vi "9_Compensate_Input_Delays_setInputDelay.vi"(8 "error in (no error)":errorcluster) -> (0 "error out":errorcluster)   [LabVIEW 2014]
uses:
  SwabianInstruments.TimeTagger
panel:
  in  "Clear Data":bool
  out "Counts per second":dbl[](array[numeric])
  in  "End Measurement":bool
  out "Rate":dbl[](array[numeric]) caption="Counts/s with delay adjustment"
  out "extracted delay [ps]\n (peak maximum)":i64
  out "Cross correlation":cluster{"getIndex":i64[], "getData":i32[]}(graph) caption="Cross correlation with compensated delay"
  out "Cross correlation without inputDelay adjustment":cluster{"getIndex":i64[], "getData":i32[]}(graph)
  # "STAGE 1\nThe internal test signal has a propagation delay between the \ndifferent input channels.\nThis example shows how to use setInputDelay to compensate the offset."
  # "STAGE 2\nThe internal test signal of channel 1 is now shifted from the measurement\nof STAGE 1 so that clicks of both channels arrive at the very same time."
  # "channel 1"
  # "channel 1"
  # "channel 2"
  # "channel 2"
  # "coincidences"
  # "coincidences"
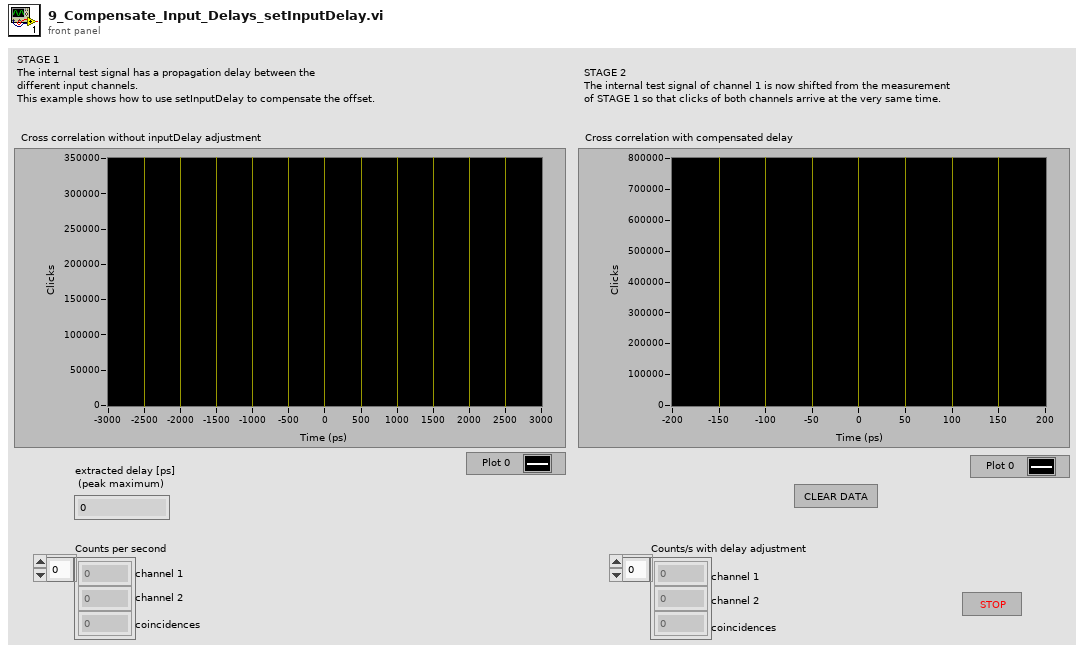
[diagram p1: front panel]
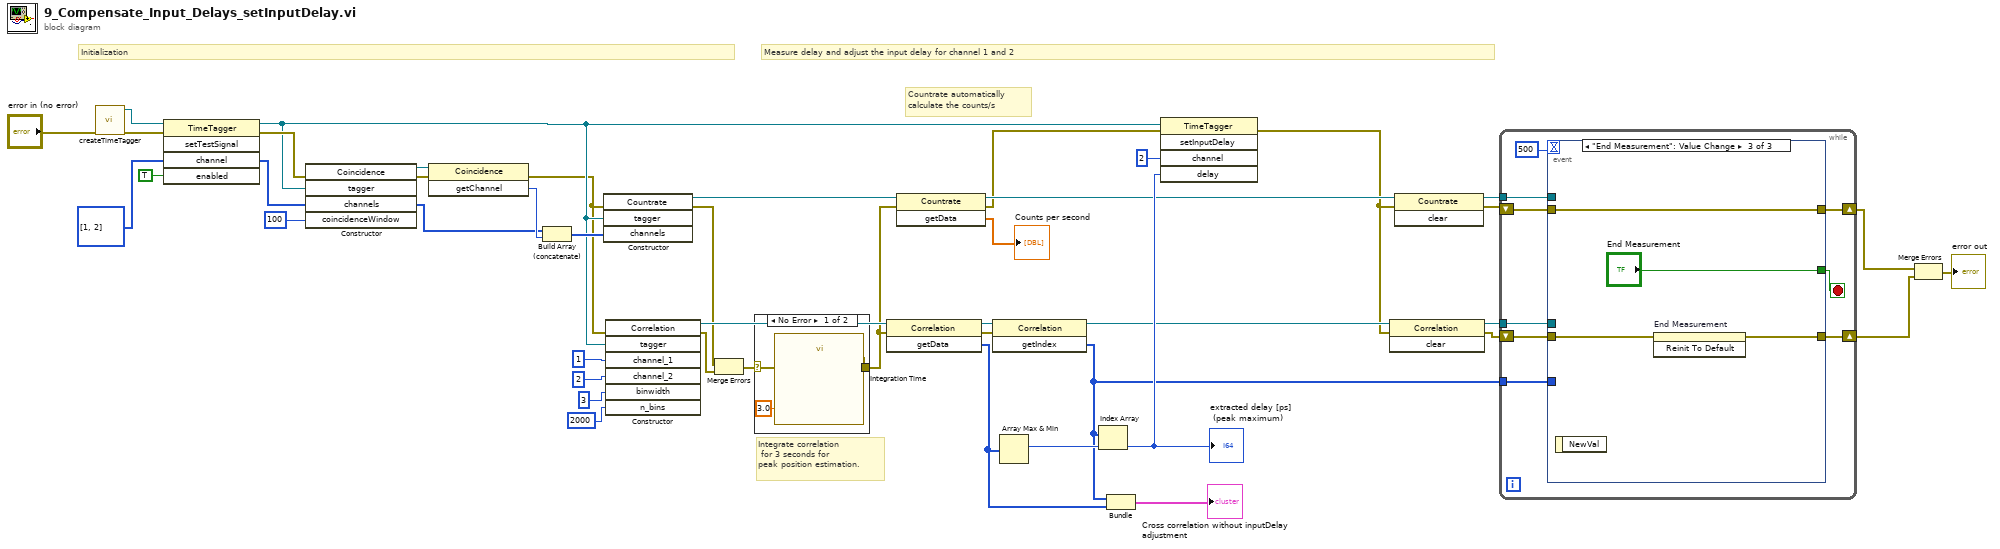
[diagram p0: block diagram]
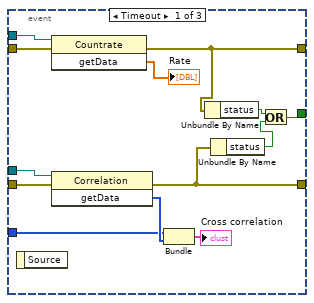
[diagram p3: hidden frame]
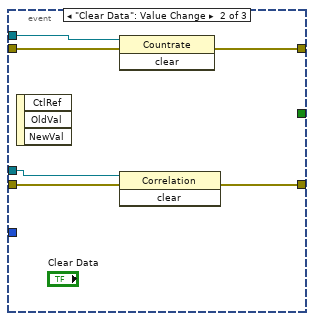
[diagram p4: hidden frame]
diagram:
  # "Integrate correlation\n for 3 seconds for\npeak position estimation."
  # "Countrate automatically \ncalculate the counts/s"
  # "Measure delay and adjust the input delay for channel 1 and 2"
  # "Initialization"
  n1 = call "createTimeTagger.vi"("error in (no error)"="error in (no error)") -> ("error out"=w19:errorcluster, "TimeTagger ref out"=w18:refnum<k24>)  [unwired: 9 in]
  n2 = invoke class="TimeTagger" method="setTestSignal"(reference=w18, error in=w19, "channel"=i32[] [1, 2], "enabled"=TRUE) -> (reference out=w7:refnum<k24>, error out=w16:errorcluster, "channel"=w13:i32[])  [unwired: 1 in, 2 out]
  n3 = constructor class="Coincidence"(error in=w16, "tagger"=w7, "channels"=w13, "coincidenceWindow"=i64 100 ("window")) -> (reference out=w22:refnum<k24>, error out=w20:errorcluster, "channels"=w14:i32[])  [unwired: 2 in, 3 out]
  n4 = invoke class="Coincidence" method="getChannel"(reference=w22, error in=w20) -> (error out=w6:errorcluster, "getChannel"=w21:i32)  [unwired: 1 in, 1 out]
  n5 = Build Array (concatenate)(w14, w21) -> (w33:i32[])
  n6 = constructor class="Countrate"(error in=w6, "tagger"=w7, "channels"=w33) -> (reference out=w26:refnum<k24>, error out=w10:errorcluster)  [unwired: 2 in, 3 out]
  n7 = constructor class="Correlation"(error in=w6, "tagger"=w7, "channel_1"=1, "channel_2"=2, "binwidth"=i64 3, "n_bins"=2000) -> (reference out=w30:refnum<k24>, error out=w9:errorcluster)  [unwired: 2 in, 6 out]
  n8 = Merge Errors(w10, w9) -> (w8:errorcluster)
  n9 = case shown="No Error" w8 {
    selector: w8 -> [w46 w49]
    tunnel: [w47 w49] -> w15
    frame No Error {
      n10 = call "Integration Time"("error in (no error)"=w46, "Delay Time (s)"=3.0) -> ("error out"=w47:errorcluster)  [unwired: 9 in]
    }
    frame Error {
    }
  }
  n11 = invoke class="Correlation" method="getData"(reference=w30, error in=w15) -> (reference out=w44:refnum<k24>, error out=w27:errorcluster, "getData"=w38:i32[])  [unwired: 1 in]
  n12 = invoke class="Countrate" method="getData"(reference=w26, error in=w15) -> (reference out=w25:refnum<k24>, error out=w23:errorcluster, "getData"=→"Counts per second":dbl[])  [unwired: 1 in]
  n13 = invoke class="Correlation" method="getIndex"(reference=w44, error in=w27) -> (reference out=w31:refnum<k24>, "getIndex"=w32:i64[])  [unwired: 1 in, 1 out]
  n14 = Array Max & Min(array=w38) -> (max index (indices)=w36:i32)  [unwired: 3 out]
  n15 = Index Array(array=w32, index=w36) -> (element=w35:i64)
  "extracted delay [ps]\n (peak maximum)" <- w35
  n16 = Bundle("getIndex"=w32, "getData"=w38) -> (→"Cross correlation without inputDelay adjustment":cluster{"getIndex":i64[], "getData":i32[]})  [unwired: 1 in]
  n17 = invoke class="TimeTagger" method="setInputDelay"(reference=w7, error in=w23, "channel"=2, "delay"=w35) -> (error out=w5:errorcluster)  [unwired: 1 in, 4 out]
  n18 = invoke class="Correlation" method="clear"(reference=w31, error in=w5) -> (reference out=w29:refnum<k24>, error out=w11:errorcluster)  [unwired: 1 in, 1 out]
  n19 = invoke class="Countrate" method="clear"(reference=w25, error in=w5) -> (reference out=w28:refnum<k24>, error out=w12:errorcluster)  [unwired: 1 in, 1 out]
  n20 = while {
    tunnel: w32 -> [w58]
    tunnel: w29 -> [w57]
    tunnel: w28 -> [w56]
    shift-right: [w53] -> w3
    shift-left: w11 -> [w55]
    shift-right: [w52] -> w4
    shift-left: w12 -> [w54]
    stop <- w51 stop-if-true
    n21 = event shown="[2] \"End Measurement\": Value Change" {
      selector: _ -> [_ _ _]
      dyn-events: _ -> [_ _ _]
      timeout: u32 500 ("milliseconds to wait") -> [_ _ _]
      tunnel: w58 -> [w70 _ _]
      tunnel: w57 -> [w68 w75 _]
      tunnel: w56 -> [w67 w77 _]
      tunnel: w55 -> [w65 w74 w79]
      tunnel: w54 -> [w64 w76 w80]
      tunnel: [w63 w73 w78] -> w53
      tunnel: [w62 w72 w80] -> w52
      tunnel: [w59 _ "End Measurement"] -> w51
      event Timeout {
        n22 = event-data() -> ()  [unwired: 1 in, 1 out]
        n23 = invoke class="Countrate" method="getData"(reference=w67, error in=w64) -> (error out=w62:errorcluster, "getData"=→"Rate":dbl[])  [unwired: 1 in, 1 out]
        n24 = invoke class="Correlation" method="getData"(reference=w68, error in=w65) -> (error out=w63:errorcluster, "getData"=w71:i32[])  [unwired: 1 in, 1 out]
        n25 = Bundle("getIndex"=w70, "getData"=w71) -> (→"Cross correlation":cluster{"getIndex":i64[], "getData":i32[]})  [unwired: 1 in]
        n26 = Unbundle By Name(w62) -> ("status"=w61:bool)
        n27 = Unbundle By Name(w63) -> ("status"=w60:bool)
        n28 = Or(x=w61, y=w60) -> (x .or. y?=w59:bool)
      }
      event "Clear Data": Value Change {
        n29 = event-data() -> ()  [unwired: 1 in, 3 out]
        n30 = invoke class="Countrate" method="clear"(reference=w77, error in=w76) -> (error out=w72:errorcluster)  [unwired: 1 in, 2 out]
        n31 = invoke class="Correlation" method="clear"(reference=w75, error in=w74) -> (error out=w73:errorcluster)  [unwired: 1 in, 2 out]
      }
      event "End Measurement": Value Change {
        n32 = event-data() -> ()  [unwired: 1 in, 1 out]
        n33 = invoke on="End Measurement" class="Bool (strict)" method="Reinit To Default"(error in=w79) -> (error out=w78:errorcluster)  [unwired: 2 in, 2 out]
      }
    }
  }
  n34 = Merge Errors(w4, w3) -> (→"error out":errorcluster)
